vi "ParametersTable.vi"(8 "error in (no error)":errorcluster, 11 "Log":refnum<vi>) -> (0 "error out":errorcluster, 3 "Cancelled?":bool)   [LabVIEW 2017]
doc: "Use this template to create a dialog box with event handling."
uses:
  Global_SNK3_HF.vi
  <vilib>/Utility/file.llb/Read Delimited Spreadsheet (DBL).vi
  <vilib>/Utility/file.llb/Write Delimited Spreadsheet (DBL).vi
panel:
  in  "OUT 2":bool
  in  "IN 2":bool
  in  "IN":bool
  in  "OUT":bool
  in  "Cancel":bool
  in  "OK":bool
  out "1D Array 4":string[](array[string])=["\"Разрешить работу ГИ №1\"", "\"№ ПЭП (с 1 по 8) подключенный к ГИ №1\"", "\"Задержка импульса ГИ №1\"", "\"Длительность импульса ГИ\"", "\"Разрешить работу приемника\"", "\"№ ПЭП (с 1 по 8) подключенный к приемнику №1\"", "\"Задержка развертки приемника №1\"", "\"Длительность развертки приемника №1\"", "\"Коэффициент усиления приемника №1\"", "\"Выходное значение ЦАП №1 управляющий коэффициентом усиления приемника №1\"", "", "", "", "", "", ""]
  out "1D Array 3":string[](array[string])=["\"Разрешить работу ГИ №1\"", "\"№ ПЭП (с 1 по 8) подключенный к ГИ №1\"", "\"Задержка импульса ГИ №1\"", "\"Длительность импульса ГИ\"", "\"Разрешить работу приемника\"", "\"№ ПЭП (с 1 по 8) подключенный к приемнику №1\"", "\"Задержка развертки приемника №1\"", "\"Длительность развертки приемника №1\"", "\"Коэффициент усиления приемника №1\"", "\"Выходное значение ЦАП №1 управляющий коэффициентом усиления приемника №1\"", "", "", "", "", "", ""]
  in  "TblParam1":sgl[][](array[numeric])=[[1.0, 2.0, 3.0, 4.0, 5.0, 6.0, 7.0, 8.0, 9.0, 10.0, 11.0, 12.0, 13.0, 14.0, 15.0, 16.0, 17.0, 18.0, 19.0, 20.0, 21.0, 22.0, 23.0, 24.0, 25.0, 26.0, 27.0, 28.0, 29.0, 30.0, 31.0, 32.0], [0.0, 0.0, 0.0, 0.0, 0.0, 0.0, 0.0, 0.0, 0.0, 0.0, 0.0, 0.0, 0.0, 0.0, 0.0, 0.0, 0.0, 0.0, 0.0, 0.0, 0.0, 0.0, 0.0, 0.0, 0.0, 0.0, 0.0, 0.0, 0.0, 0.0, 0.0, 0.0], [0.0, 0.0, 0.0, 0.0, 0.0, 0.0, 0.0, 0.0, 0.0, 0.0, 0.0, 0.0, 0.0, 0.0, 0.0, 0.0, 0.0, 0.0, 0.0, 0.0, 0.0, 0.0, 0.0, 0.0, 0.0, 0.0, 0.0, 0.0, 0.0, 0.0, 0.0, 0.0], [0.0, 0.0, 0.0, 0.0, 0.0, 0.0, 0.0, 0.0, 0.0, 0.0, 0.0, 0.0, 0.0, 0.0, 0.0, 0.0, 0.0, 0.0, 0.0, 0.0, 0.0, 0.0, 0.0, 0.0, 0.0, 0.0, 0.0, 0.0, 0.0, 0.0, 0.0, 0.0], [0.0, 0.0, 0.0, 0.0, 0.0, 0.0, 0.0, 0.0, 0.0, 0.0, 0.0, 0.0, 0.0, 0.0, 0.0, 0.0, 0.0, 0.0, 0.0, 0.0, 0.0, 0.0, 0.0, 0.0, 0.0, 0.0, 0.0, 0.0, 0.0, 0.0, 0.0, 0.0], [0.0, 0.0, 0.0, 0.0, 0.0, 0.0, 0.0, 0.0, 0.0, 0.0, 0.0, 0.0, 0.0, 0.0, 0.0, 0.0, 0.0, 0.0, 0.0, 0.0, 0.0, 0.0, 0.0, 0.0, 0.0, 0.0, 0.0, 0.0, 0.0, 0.0, 0.0, 0.0], [0.0, 0.0, 0.0, 0.0, 0.0, 0.0, 0.0, 0.0, 0.0, 0.0, 0.0, 0.0, 0.0, 0.0, 0.0, 0.0, 0.0, 0.0, 0.0, 0.0, 0.0, 0.0, 0.0, 0.0, 0.0, 0.0, 0.0, 0.0, 0.0, 0.0, 0.0, 0.0], [0.0, 0.0, 0.0, 0.0, 0.0, 0.0, 0.0, 0.0, 0.0, 0.0, 0.0, 0.0, 0.0, 0.0, 0.0, 0.0, 0.0, 0.0, 0.0, 0.0, 0.0, 0.0, 0.0, 0.0, 0.0, 0.0, 0.0, 0.0, 0.0, 0.0, 0.0, 0.0], [0.0, 0.0, 0.0, 0.0, 0.0, 0.0, 0.0, 0.0, 0.0, 0.0, 0.0, 0.0, 0.0, 0.0, 0.0, 0.0, 0.0, 0.0, 0.0, 0.0, 0.0, 0.0, 0.0, 0.0, 0.0, 0.0, 0.0, 0.0, 0.0, 0.0, 0.0, 0.0], [0.0, 0.0, 0.0, 0.0, 0.0, 0.0, 0.0, 0.0, 0.0, 0.0, 0.0, 0.0, 0.0, 0.0, 0.0, 0.0, 0.0, 0.0, 0.0, 0.0, 0.0, 0.0, 0.0, 0.0, 0.0, 0.0, 0.0, 0.0, 0.0, 0.0, 0.0, 0.0], [0.0, 0.0, 0.0, 0.0, 0.0, 0.0, 0.0, 0.0, 0.0, 0.0, 0.0, 0.0, 0.0, 0.0, 0.0, 0.0, 0.0, 0.0, 0.0, 0.0, 0.0, 0.0, 0.0, 0.0, 0.0, 0.0, 0.0, 0.0, 0.0, 0.0, 0.0, 0.0]]
  in  "TblParam0":sgl[][](array[numeric])=[[1.0, 2.0, 3.0, 4.0, 5.0, 6.0, 7.0, 8.0, 9.0, 10.0, 11.0, 12.0, 13.0, 14.0, 15.0, 16.0, 17.0, 18.0, 19.0, 20.0, 21.0, 22.0, 23.0, 24.0, 25.0, 26.0, 27.0, 28.0, 29.0, 30.0, 31.0, 32.0], [0.0, 0.0, 0.0, 0.0, 0.0, 0.0, 0.0, 0.0, 0.0, 0.0, 0.0, 0.0, 0.0, 0.0, 0.0, 0.0, 0.0, 0.0, 0.0, 0.0, 0.0, 0.0, 0.0, 0.0, 0.0, 0.0, 0.0, 0.0, 0.0, 0.0, 0.0, 0.0], [0.0, 0.0, 0.0, 0.0, 0.0, 0.0, 0.0, 0.0, 0.0, 0.0, 0.0, 0.0, 0.0, 0.0, 0.0, 0.0, 0.0, 0.0, 0.0, 0.0, 0.0, 0.0, 0.0, 0.0, 0.0, 0.0, 0.0, 0.0, 0.0, 0.0, 0.0, 0.0], [0.0, 0.0, 0.0, 0.0, 0.0, 0.0, 0.0, 0.0, 0.0, 0.0, 0.0, 0.0, 0.0, 0.0, 0.0, 0.0, 0.0, 0.0, 0.0, 0.0, 0.0, 0.0, 0.0, 0.0, 0.0, 0.0, 0.0, 0.0, 0.0, 0.0, 0.0, 0.0], [0.0, 0.0, 0.0, 0.0, 0.0, 0.0, 0.0, 0.0, 0.0, 0.0, 0.0, 0.0, 0.0, 0.0, 0.0, 0.0, 0.0, 0.0, 0.0, 0.0, 0.0, 0.0, 0.0, 0.0, 0.0, 0.0, 0.0, 0.0, 0.0, 0.0, 0.0, 0.0], [0.0, 0.0, 0.0, 0.0, 0.0, 0.0, 0.0, 0.0, 0.0, 0.0, 0.0, 0.0, 0.0, 0.0, 0.0, 0.0, 0.0, 0.0, 0.0, 0.0, 0.0, 0.0, 0.0, 0.0, 0.0, 0.0, 0.0, 0.0, 0.0, 0.0, 0.0, 0.0], [0.0, 0.0, 0.0, 0.0, 0.0, 0.0, 0.0, 0.0, 0.0, 0.0, 0.0, 0.0, 0.0, 0.0, 0.0, 0.0, 0.0, 0.0, 0.0, 0.0, 0.0, 0.0, 0.0, 0.0, 0.0, 0.0, 0.0, 0.0, 0.0, 0.0, 0.0, 0.0], [0.0, 0.0, 0.0, 0.0, 0.0, 0.0, 0.0, 0.0, 0.0, 0.0, 0.0, 0.0, 0.0, 0.0, 0.0, 0.0, 0.0, 0.0, 0.0, 0.0, 0.0, 0.0, 0.0, 0.0, 0.0, 0.0, 0.0, 0.0, 0.0, 0.0, 0.0, 0.0], [0.0, 0.0, 0.0, 0.0, 0.0, 0.0, 0.0, 0.0, 0.0, 0.0, 0.0, 0.0, 0.0, 0.0, 0.0, 0.0, 0.0, 0.0, 0.0, 0.0, 0.0, 0.0, 0.0, 0.0, 0.0, 0.0, 0.0, 0.0, 0.0, 0.0, 0.0, 0.0], [0.0, 0.0, 0.0, 0.0, 0.0, 0.0, 0.0, 0.0, 0.0, 0.0, 0.0, 0.0, 0.0, 0.0, 0.0, 0.0, 0.0, 0.0, 0.0, 0.0, 0.0, 0.0, 0.0, 0.0, 0.0, 0.0, 0.0, 0.0, 0.0, 0.0, 0.0, 0.0], [0.0, 0.0, 0.0, 0.0, 0.0, 0.0, 0.0, 0.0, 0.0, 0.0, 0.0, 0.0, 0.0, 0.0, 0.0, 0.0, 0.0, 0.0, 0.0, 0.0, 0.0, 0.0, 0.0, 0.0, 0.0, 0.0, 0.0, 0.0, 0.0, 0.0, 0.0, 0.0]]
  # "Параметры цикла для ПЭП 1...8"
  # "Параметры цикла для ПЭП 9...16"
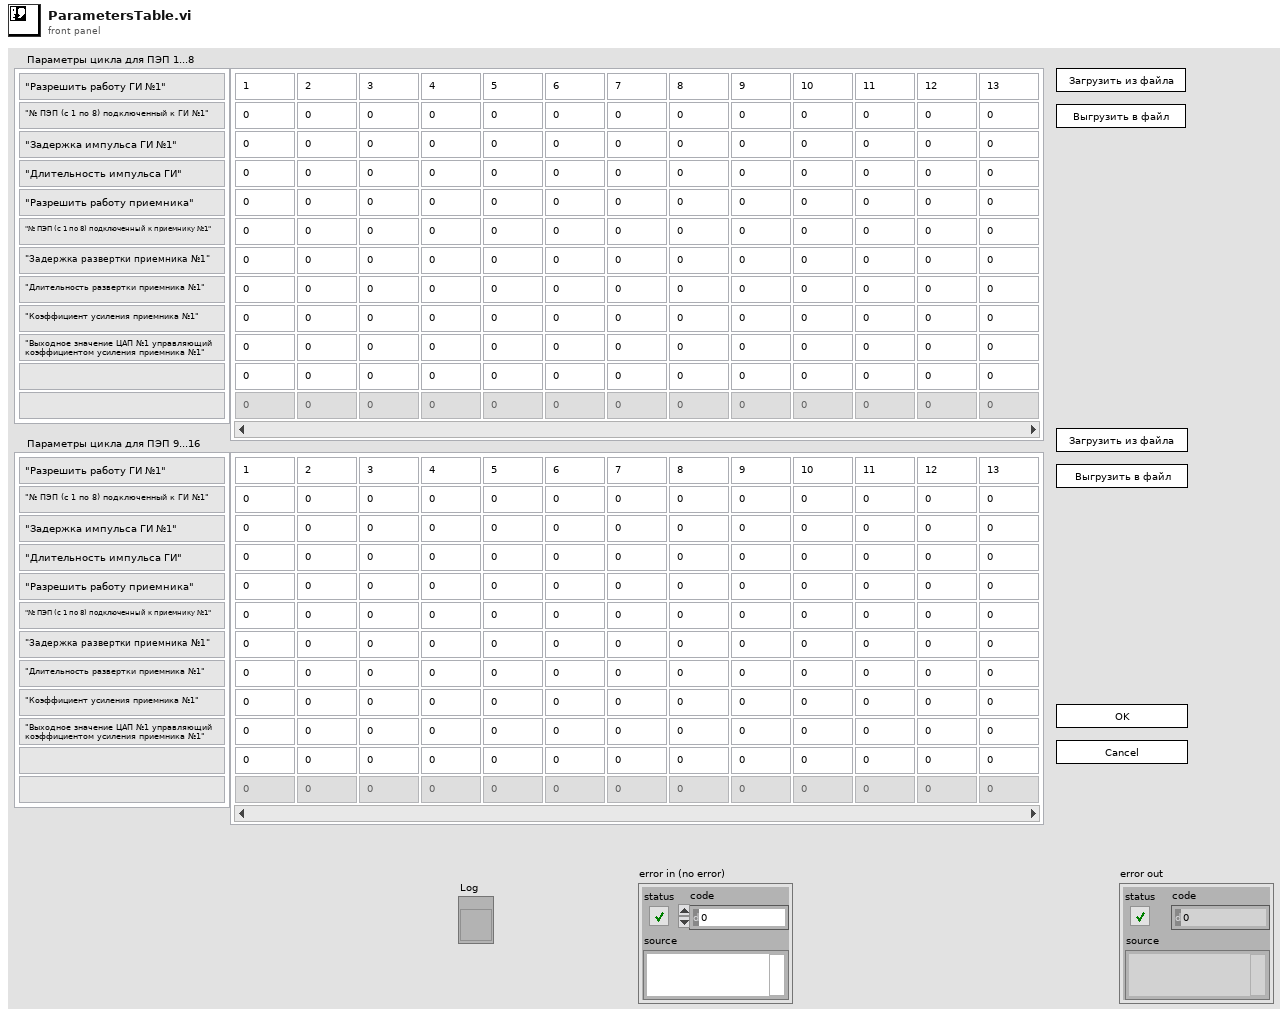
[diagram p1: front panel]
types:
  T1 = typedef "LV_Unicorn.lvlib/unicorn_Param.ctl" = cluster{"conParam":T2, "Param":T3}
  T2 = typedef "LV_Unicorn.lvlib/unicorn_conn.ctl" = cluster{"ReadIntParam":bool, "ReadDescrParam":bool, "ReadFloatParam":bool, "debug":bool, "ReadJSON":bool, "IP_address":string, "N_attempts":i32, "type_con":enum16{"Serial", "TCP"}, "MB_address":i32, "VISA":refnum<visa-resource-name>, "connection ID":refnum<k5>, "nameDevices":string, "timeout":i32, "port":u16, "type_version":string, "baud_rate":u32, "VersionControl":bool, "TCP_conn":bool, "WindowSize":i32}
  T3 = typedef "LV_Unicorn.lvlib/unicorn_JSON.ctl" = cluster{"NumParam":cluster{"NTelem":i32, "NInt":i32, "NFloat":i32, "NTable":i32}, "ParamInt":T4, "Telemetry":T5, "Table":T6, "ParamFloat":T7}
  T4 = typedef "LV_Unicorn.lvlib/unicorn_ParamInt.ctl" = cluster{"ID":string, "Num":i32, "Name":string, "Type":string, "Enum":string, "Desc":string, "Unit":string, "Access":string, "FormatStr":string, "Min":i32, "Max":i32}[]
  T5 = typedef "LV_Unicorn.lvlib/unicorn_Telemetry.ctl" = cluster{"ID":string, "Num":i32, "Name":string, "Desc":string, "Unit":string, "FormatStr":string, "Min":i32, "Max":i32}[]
  T6 = typedef "LV_Unicorn.lvlib/unicorn_Table.ctl" = cluster{"Num":i32, "Access":string, "ColumnCount":i32, "NeedParamPrepare":bool, "Columns":cluster{"Column":i32, "Desc":string, "Name":string}[], "DataType":string, "FormatStr":string, "ID":string, "Name":string, "RowCount":i32, "Rows":cluster{"Desc":string, "ID":string, "Max":i32, "Min":i32, "Name":string, "Row":i32, "Unit":string}[], "Type":string}[]
  T7 = typedef "LV_Unicorn.lvlib/unicorn_ParamFloat.ctl" = cluster{"ID":string, "Num":i32, "Name":string, "Type":string, "Enum":string, "Desc":string, "Unit":string, "Access":string, "FormatStr":string, "Min":sgl, "Max":sgl}[]
  T8 = cluster{"Num":i32, "Access":string, "ColumnCount":i32, "NeedParamPrepare":bool, "Columns":cluster{"Column":i32, "Desc":string, "Name":string}[], "DataType":string, "FormatStr":string, "ID":string, "Name":string, "RowCount":i32, "Rows":cluster{"Desc":string, "ID":string, "Max":i32, "Min":i32, "Name":string, "Row":i32, "Unit":string}[], "Type":string}
  T9 = cluster{"Desc":string, "ID":string, "Max":i32, "Min":i32, "Name":string, "Row":i32, "Unit":string}[]
  T10 = typedef "LVRectTypeDef.ctl" = cluster{"Left":i16, "Top":i16, "Right":i16, "Bottom":i16}
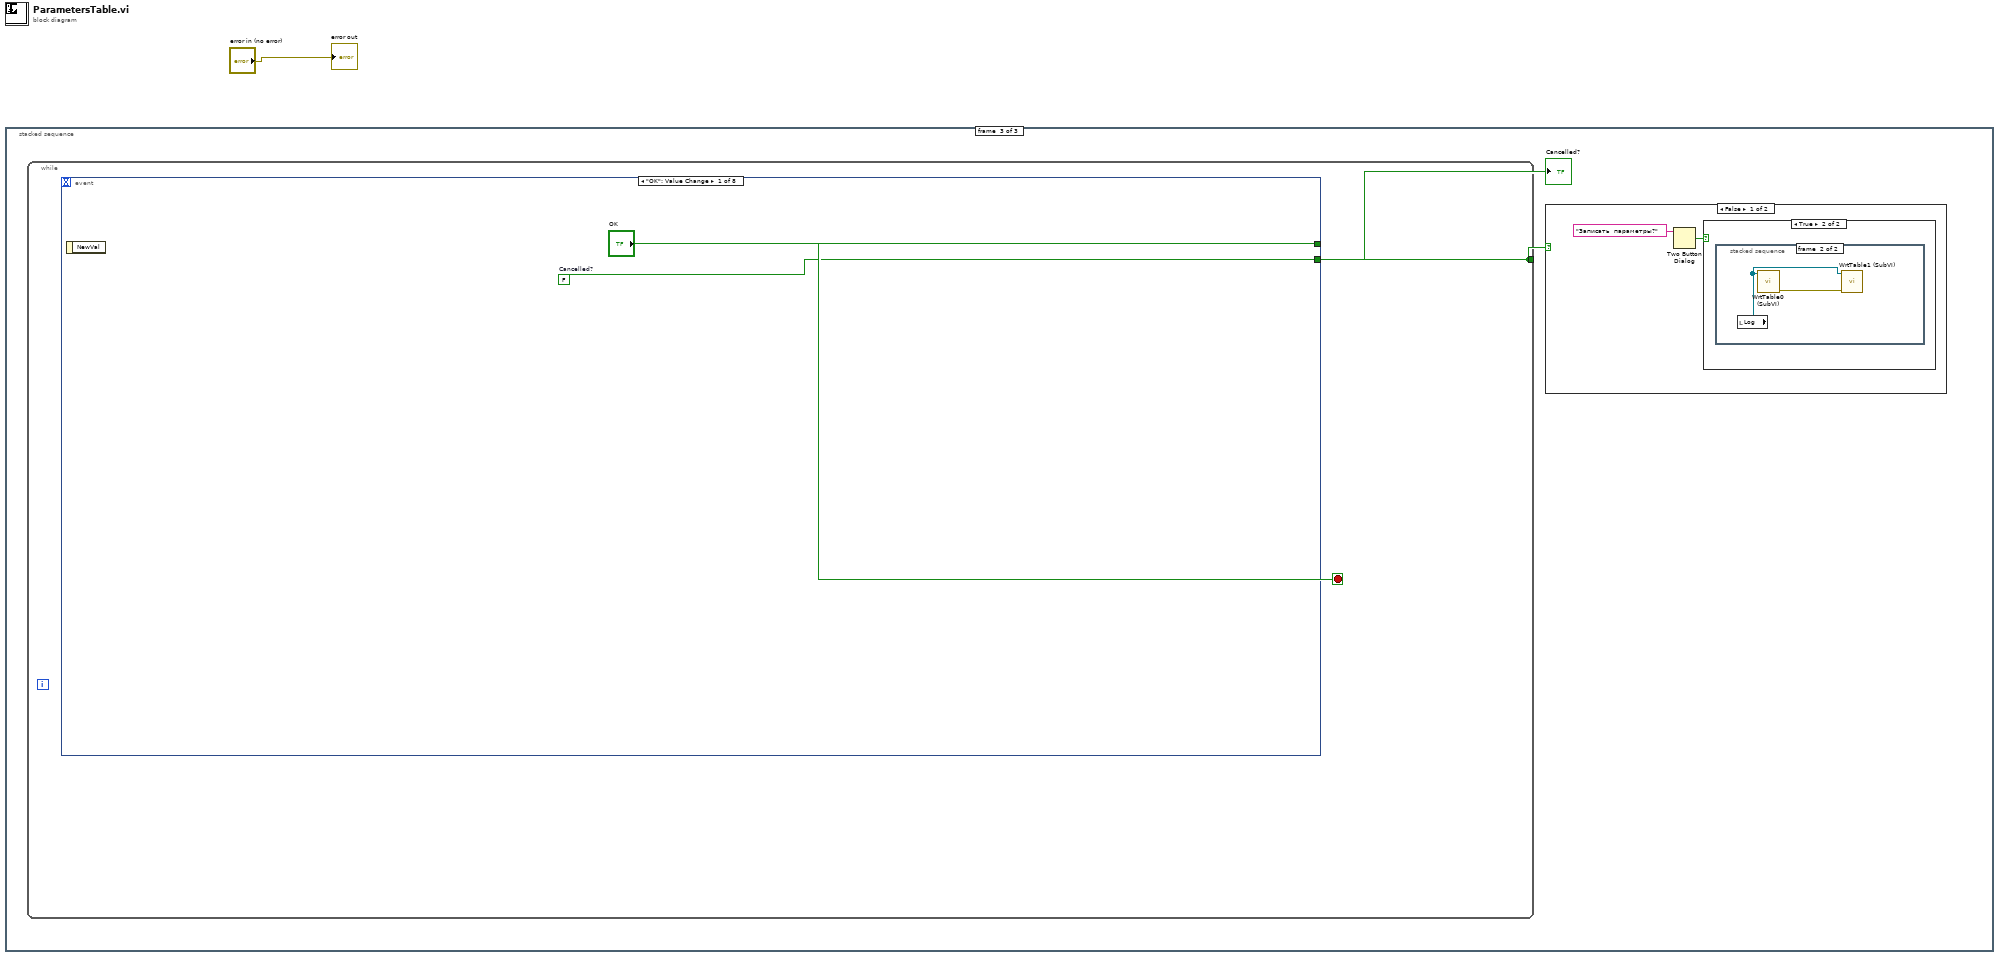
[diagram p0: block diagram]
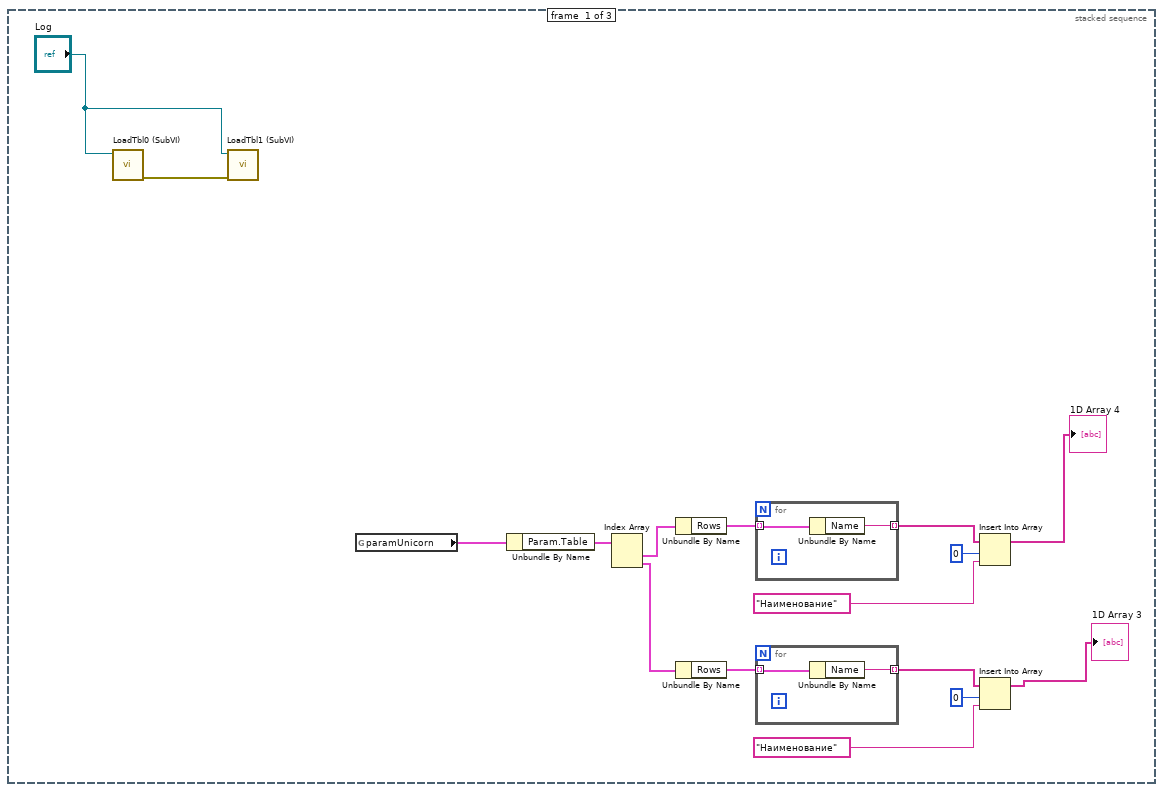
[diagram p2: hidden frame]
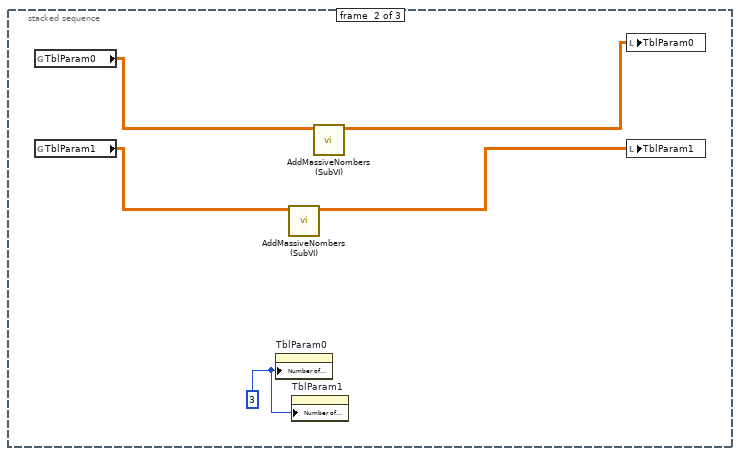
[diagram p3: hidden frame]
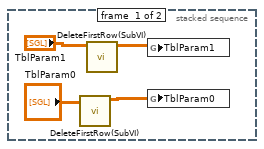
[diagram p5: hidden frame]
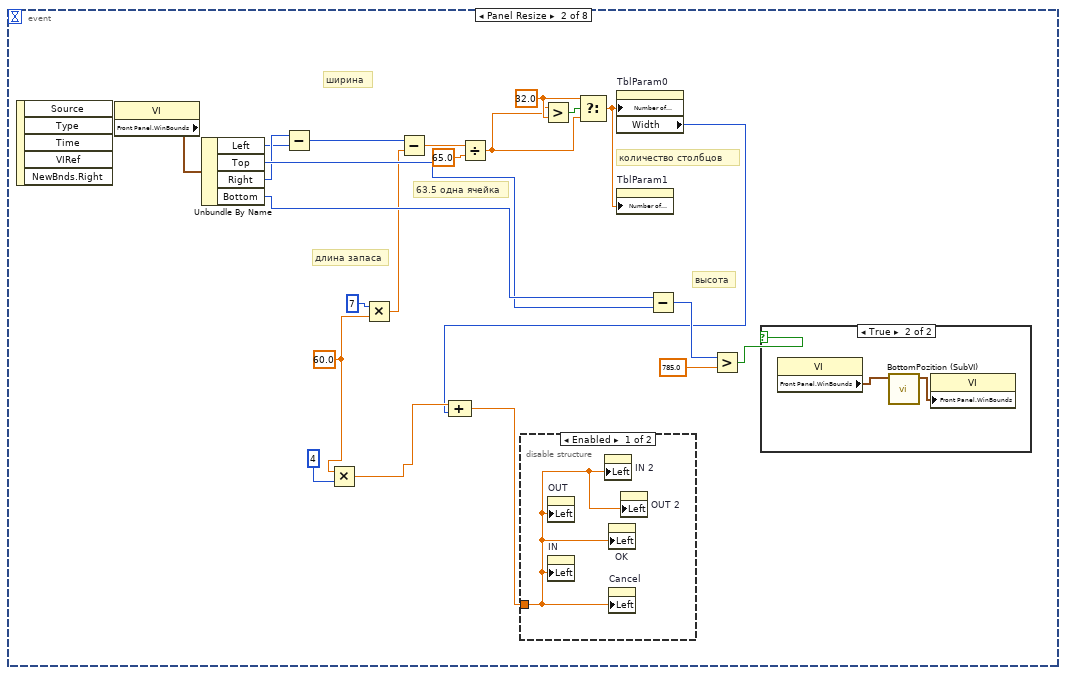
[diagram p7: hidden frame]
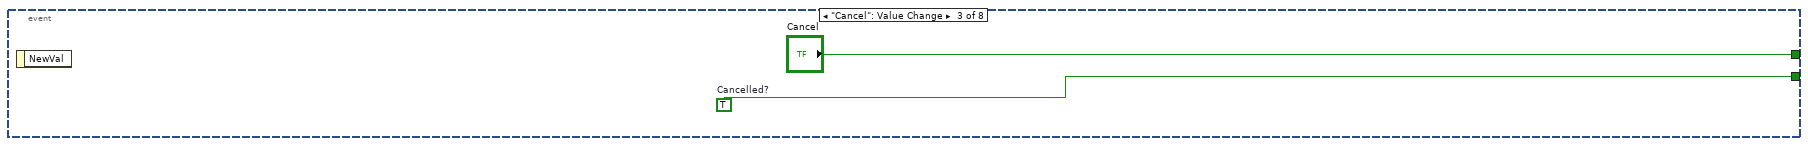
[diagram p10: hidden frame]
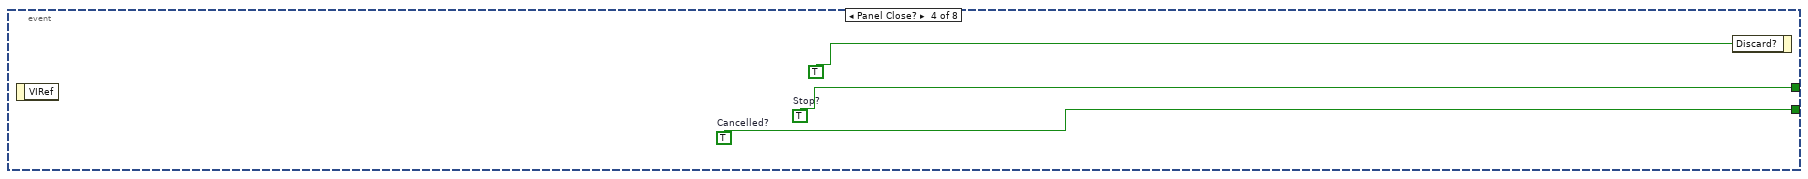
[diagram p11: hidden frame]
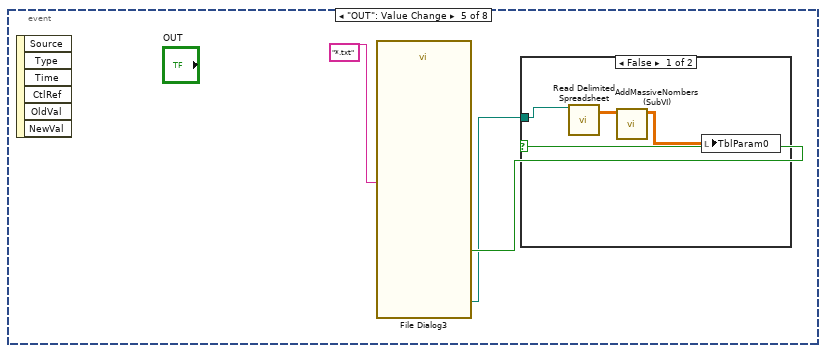
[diagram p12: hidden frame]
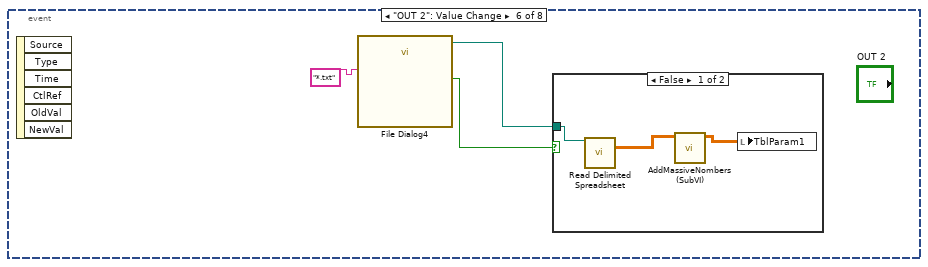
[diagram p14: hidden frame]
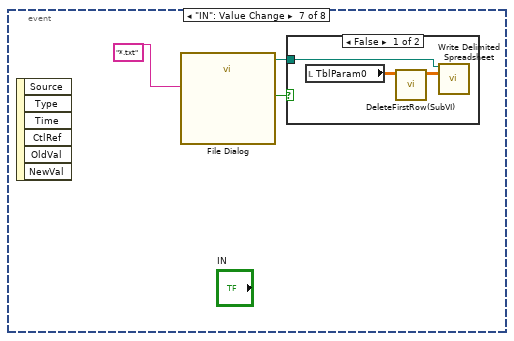
[diagram p16: hidden frame]
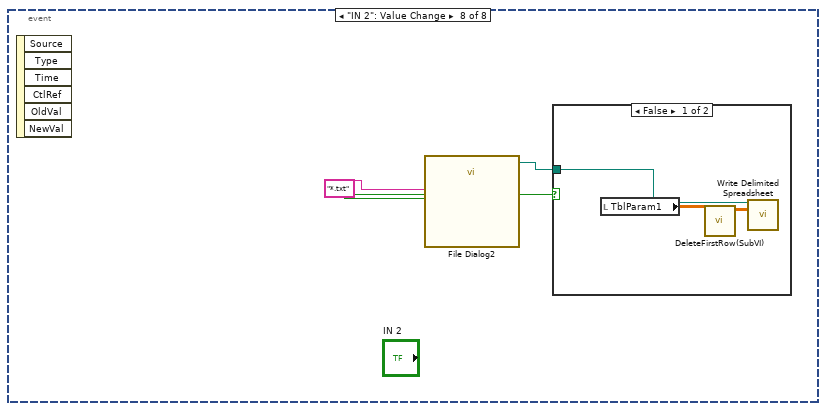
[diagram p18: hidden frame]
diagram:
  n1 = stacked-sequence {
    frame #0 {
      n2 = call "LoadTbl0 (SubVI).vi"("Log"="Log") -> ("error out"=w17:errorcluster)  [unwired: 10 in]
      n3 = call "LoadTbl1 (SubVI).vi"("error in"=w17, "Log"="Log") -> ()  [unwired: 9 in, 1 out]
      n4 = global read "Global_SNK3_HF.vi" "paramUnicorn"() -> (w15:T1)
      n5 = Unbundle By Name(w15) -> ("Param.Table"=w13:T6)
      n6 = Index Array(array=w13) -> (element #1=w12:T8, element #2=w3:T8)  [unwired: 2 in]
      n7 = Unbundle By Name(w12) -> ("Rows"=w11:T9)
      n8 = Unbundle By Name(w3) -> ("Rows"=w5:T9)
      n9 = for {
        tunnel: w11 -> [w21] mode=indexing
        tunnel: [w20] -> w9 mode=indexing
        n10 = Unbundle By Name(w21) -> ("Name"=w20:string)
      }
      n11 = for {
        tunnel: w5 -> [w19] mode=indexing
        tunnel: [w18] -> w7 mode=indexing
        n12 = Unbundle By Name(w19) -> ("Name"=w18:string)
      }
      n13 = Insert Into Array(array=w9, index=0, new element="Наименование") -> (→"1D Array 4":string[])
      n14 = Insert Into Array(array=w7, index=0, new element="Наименование") -> (→"1D Array 3":string[])
    }
    frame #1 {
      w22 = u32 3 ("Number of Columns")
      n15 = global read "Global_SNK3_HF.vi" "TblParam0"() -> (w26:sgl[][])
      n16 = global read "Global_SNK3_HF.vi" "TblParam1"() -> (w24:sgl[][])
      n17 = property on="TblParam0" class="Arr (strict)"("Number of Columns"=w22) -> ()  [unwired: 2 in, 2 out]
      n18 = call "AddMassiveNombers (SubVI).vi"("TblParam in"=w24) -> ("TblParam out"=w23:sgl[][])  [unwired: 10 in]
      n19 = property on="TblParam1" class="Arr (strict)"("Number of Columns"=w22) -> ()  [unwired: 2 in, 2 out]
      n20 = call "AddMassiveNombers (SubVI).vi"("TblParam in"=w26) -> ("TblParam out"=w25:sgl[][])  [unwired: 10 in]
      n21 = local write "TblParam0"(w25) -> ()
      n22 = local write "TblParam1"(w23) -> ()
    }
    frame #2 {
      n23 = while {
        tunnel: [w36] -> w27
        stop <- w37 stop-if-true
        n24 = event shown="[0] \"OK\": Value Change" {
          selector: _ -> [_ _ _ _ _ _ _ _]
          dyn-events: _ -> [_ _ _ _ _ _ _ _]
          timeout: _ -> [_ _ _ _ _ _ _ _]
          tunnel: ["OK" _ "Cancel" w68 _ _ _ _] -> w37
          tunnel: [w39 _ w66 w67 _ _ _ _] -> w36
          event "OK": Value Change {
            w39 = FALSE  # Cancelled?
            n25 = event-data() -> ()  [unwired: 1 in, 1 out]
          }
          event Panel Resize {
            w44 = 32.0 ("y")
            w49 = 60.0 ("y")
            # "высота"
            # "количество столбцов"
            # "длина запаса"
            # "ширина"
            # "63.5 одна ячейка"
            n26 = event-data() -> ()  [unwired: 1 in, 5 out]
            n27 = property class="VI"() -> ("Front Panel.WinBounds"=w61:T10)  [unwired: 2 in, 2 out]
            n28 = Unbundle By Name(w61) -> ("Left"=w41:i16, "Top"=w53:i16, "Right"=w52:i16, "Bottom"=w55:i16)
            n29 = Subtract(x=w52, y=w41) -> (x-y=w58:i16)
            n30 = Multiply(x=w49, y=4) -> (x*y=w48:dbl)
            n31 = Multiply(x=7, y=w49) -> (x*y=w51:dbl)
            n32 = Subtract(x=w58, y=w51) -> (x-y=w50:dbl)
            n33 = Divide(x=w50, y=65.0) -> (x/y=w43:dbl)
            n34 = Greater?(x=w43, y=w44) -> (0:w45:bool)
            n35 = Select(t=w44, s=w45, f=w43) -> (s? t:f=w42:dbl)
            n36 = property on="TblParam0" class="Arr (strict)"("Number of Columns"=w42) -> ("Width"=w46:u32)  [unwired: 2 in, 2 out]
            n37 = Compound Arithmetic op=unknown(w48, w46) -> (w40:dbl)
            n38 = disable-structure shown="Enabled" {
              disable-tunnel: w40 -> [w62 _]
              frame Enabled {
                n39 = property on="OUT" class="Bool"("Left"=w62) -> ()  [unwired: 2 in, 2 out]
                n40 = property on="IN" class="Bool"("Left"=w62) -> ()  [unwired: 2 in, 2 out]
                n41 = property on="IN 2" class="Bool"("Left"=w62) -> ()  [unwired: 2 in, 2 out]
                n42 = property on="OK" class="Bool"("Left"=w62) -> ()  [unwired: 2 in, 2 out]
                n43 = property on="Cancel" class="Bool"("Left"=w62) -> ()  [unwired: 2 in, 2 out]
                n44 = property on="OUT 2" class="Bool"("Left"=w62) -> ()  [unwired: 2 in, 2 out]
              }
              frame Disabled {
              }
            }
            n45 = property on="TblParam1" class="Arr (strict)"("Number of Columns"=w42) -> ()  [unwired: 2 in, 2 out]
            n46 = Subtract(x=w55, y=w53) -> (x-y=w57:i16)
            n47 = Greater?(x=w57, y=785.0) -> (0:w56:bool)
            n48 = case shown="True" w56 {
              frame False {
              }
              frame True {
                n49 = property class="VI"() -> ("Front Panel.WinBounds"=w63:T10)  [unwired: 2 in, 2 out]
                n50 = call "BottomPozition (SubVI).vi"("Front Panel Window:Window Bounds"=w63) -> ("Front Panel Window:Window Bounds 2"=w64:T10)  [unwired: 10 in]
                n51 = property class="VI"("Front Panel.WinBounds"=w64) -> ()  [unwired: 2 in, 2 out]
              }
            }
          }
          event "Cancel": Value Change {
            w66 = TRUE  # Cancelled?
            n52 = event-data() -> ()  [unwired: 1 in, 1 out]
          }
          event Panel Close? {
            w67 = TRUE  # Cancelled?
            w68 = TRUE  # Stop?
            n53 = event-data() -> ()  [unwired: 1 in, 1 out]
            n54 = event-data("Discard?"=TRUE) -> ()  [unwired: 1 in, 1 out]
          }
          event "OUT": Value Change {
            n55 = event-data() -> ()  [unwired: 1 in, 6 out]
            n56 = call "File Dialog3"("pattern (all files)"="*.txt") -> ("selected path"=w71:path, "cancelled"=w72:bool)  [unwired: 11 in, 2 out]
            n57 = case shown="False" w72 {
              tunnel: w71 -> [w73 _]
              frame False {
                n58 = call-poly <vilib>:"Read Delimited Spreadsheet.vi"("file path (dialog if empty)"=w73) -> ("all rows"=w74:dbl[][])  [unwired: 9 in, 5 out]
                n59 = call "AddMassiveNombers (SubVI).vi"("TblParam in"=w74) -> ("TblParam out"=w75:sgl[][])  [unwired: 10 in]
                n60 = local write "TblParam0"(w75) -> ()
              }
              frame True {
              }
            }
          }
          event "OUT 2": Value Change {
            n61 = event-data() -> ()  [unwired: 1 in, 6 out]
            n62 = call "File Dialog4"("pattern (all files)"="*.txt") -> ("selected path"=w78:path, "cancelled"=w77:bool)  [unwired: 11 in, 2 out]
            n63 = case shown="False" w77 {
              tunnel: w78 -> [w79 _]
              frame False {
                n64 = call-poly <vilib>:"Read Delimited Spreadsheet.vi"("file path (dialog if empty)"=w79) -> ("all rows"=w80:dbl[][])  [unwired: 9 in, 5 out]
                n65 = call "AddMassiveNombers (SubVI).vi"("TblParam in"=w80) -> ("TblParam out"=w81:sgl[][])  [unwired: 10 in]
                n66 = local write "TblParam1"(w81) -> ()
              }
              frame True {
              }
            }
          }
          event "IN": Value Change {
            n67 = event-data() -> ()  [unwired: 1 in, 6 out]
            n68 = call "File Dialog"("pattern (all files)"="*.txt") -> ("selected path"=w83:path, "cancelled"=w84:bool)  [unwired: 11 in, 2 out]
            n69 = case shown="False" w84 {
              tunnel: w83 -> [w85 _]
              frame False {
                n70 = local read "TblParam0"() -> (w86:sgl[][])
                n71 = call "DeleteFirstRow(SubVI).vi"("TblParam in"=w86) -> ("TblParam out"=w87:sgl[][])  [unwired: 10 in]
                n72 = call-poly <vilib>:"Write Delimited Spreadsheet.vi"("file path (dialog if empty)"=w85, "2D data"=w87) -> ()  [unwired: 12 in, 2 out]
              }
              frame True {
              }
            }
          }
          event "IN 2": Value Change {
            n73 = event-data() -> ()  [unwired: 1 in, 6 out]
            n74 = call "File Dialog2"("pattern (all files)"="*.txt") -> ("selected path"=w89:path, "cancelled"=w90:bool)  [unwired: 11 in, 2 out]
            n75 = case shown="False" w90 {
              tunnel: w89 -> [w91 _]
              frame False {
                n76 = local read "TblParam1"() -> (w92:sgl[][])
                n77 = call "DeleteFirstRow(SubVI).vi"("TblParam in"=w92) -> ("TblParam out"=w93:sgl[][])  [unwired: 10 in]
                n78 = call-poly <vilib>:"Write Delimited Spreadsheet.vi"("file path (dialog if empty)"=w91, "2D data"=w93) -> ()  [unwired: 12 in, 2 out]
              }
              frame True {
              }
            }
          }
        }
      }
      "Cancelled?" <- w27
      n79 = case shown="False" w27 {
        frame False {
          n80 = Two Button Dialog(message="Записать  параметры?") -> (T button?=w29:bool)  [unwired: 2 in]
          n81 = case shown="True" w29 {
            frame False {
            }
            frame True {
              n82 = stacked-sequence {
                frame #0 {
                  n83 = call "DeleteFirstRow(SubVI).vi"("TblParam in"="TblParam0") -> ("TblParam out"=w30:sgl[][])  [unwired: 10 in]
                  n84 = call "DeleteFirstRow(SubVI).vi"("TblParam in"="TblParam1") -> ("TblParam out"=w32:sgl[][])  [unwired: 10 in]
                  n85 = global write "Global_SNK3_HF.vi" "TblParam1"(w32) -> ()
                  n86 = global write "Global_SNK3_HF.vi" "TblParam0"(w30) -> ()
                }
                frame #1 {
                  n87 = local read "Log"() -> (w34:refnum<vi>)
                  n88 = call "WrtTable0 (SubVI).vi"("Log"=w34) -> ("error out"=w35:errorcluster)  [unwired: 10 in]
                  n89 = call "WrtTable1 (SubVI).vi"("error in"=w35, "Log"=w34) -> ()  [unwired: 9 in, 1 out]
                }
              }
            }
          }
        }
        frame True {
        }
      }
    }
  }
  "error out" <- "error in (no error)"
